vi "combinational-logic-7-segment-origional.vi"(8 "4-bit-reg-input":T1) -> (0 "4-bit-reg-output":T1, 3 "7-segment CTRL out":T2)   [LabVIEW 2021]
uses:
  4-bit-disp.ctl
  7-segment-display.ctl
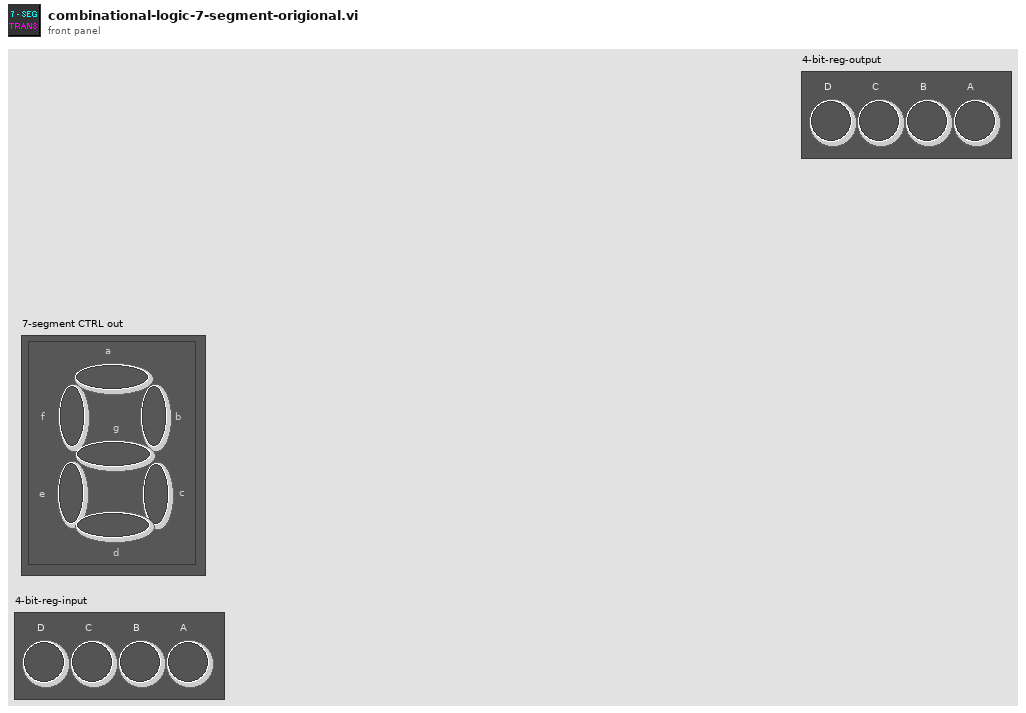
[diagram p1: front panel]
types:
  T1 = typedef "4-bit-disp.ctl" = cluster{"D":bool, "C":bool, "B":bool, "A":bool}
  T2 = typedef "7-segment-display.ctl" = cluster{"a":bool, "b":bool, "c":bool, "d":bool, "e":bool, "f":bool, "g":bool}
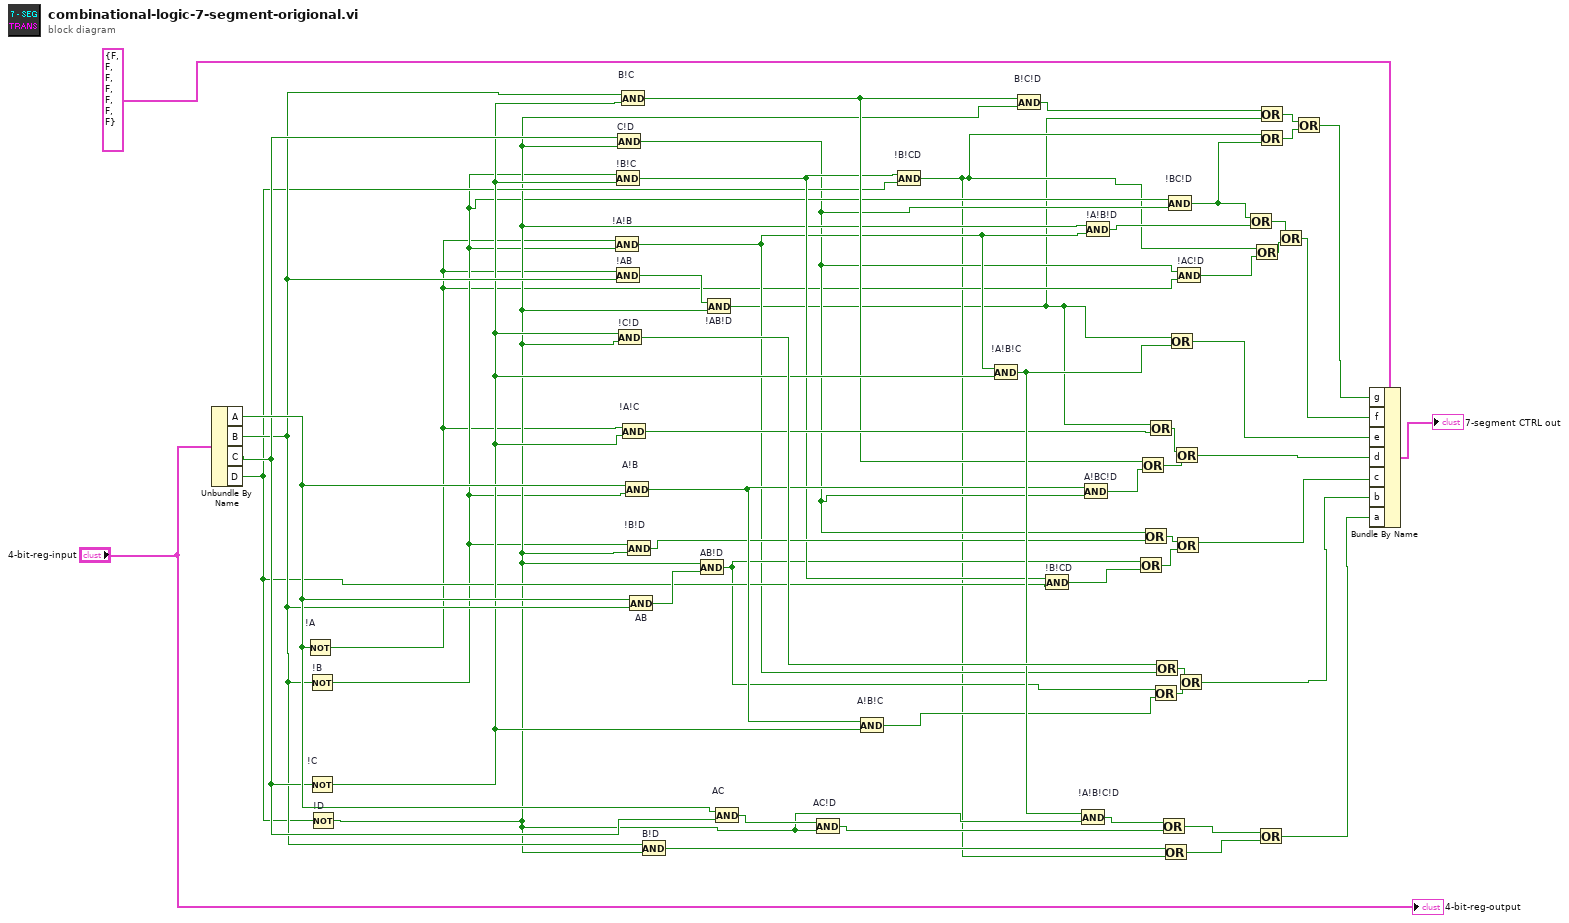
[diagram p0: block diagram]
diagram:
  n1 = Unbundle By Name("4-bit-reg-input") -> ("A"=w36:bool, "B"=w30:bool, "C"=w35:bool, "D"=w19:bool)
  n2 = Not "!A"(x=w36) -> (.not. x?=w7:bool)
  n3 = Not "!B"(x=w30) -> (.not. x?=w10:bool)
  n4 = Not "!C"(x=w35) -> (.not. x?=w28:bool)
  n5 = Not "!D"(x=w19) -> (.not. x?=w12:bool)
  n6 = And "!A!B"(x=w7, y=w10) -> (x .and. y?=w13:bool)
  n7 = And "!B!C"(x=w10, y=w28) -> (x .and. y?=w20:bool)
  n8 = And "!AB"(x=w7, y=w30) -> (x .and. y?=w47:bool)
  n9 = And "C!D"(x=w35, y=w12) -> (x .and. y?=w8:bool)
  n10 = And "!C!D"(x=w28, y=w12) -> (x .and. y?=w38:bool)
  n11 = And "B!C"(x=w30, y=w28) -> (x .and. y?=w26:bool)
  n12 = And "!A!C"(x=w7, y=w28) -> (x .and. y?=w29:bool)
  n13 = And "A!B"(x=w36, y=w10) -> (x .and. y?=w24:bool)
  n14 = And "!B!D"(x=w10, y=w12) -> (x .and. y?=w22:bool)
  n15 = And "AB"(x=w36, y=w30) -> (x .and. y?=w21:bool)
  n16 = And "B!D"(x=w30, y=w12) -> (x .and. y?=w37:bool)
  n17 = And "AB!D"(x=w12, y=w21) -> (x .and. y?=w16:bool)
  n18 = And "!AB!D"(x=w47, y=w12) -> (x .and. y?=w1:bool)
  n19 = And "AC"(x=w36, y=w35) -> (x .and. y?=w33:bool)
  n20 = And "AC!D"(x=w33, y=w12) -> (x .and. y?=w34:bool)
  n21 = And "A!B!C"(x=w24, y=w28) -> (x .and. y?=w15:bool)
  n22 = And "!B!CD"(x=w20, y=w19) -> (x .and. y?=w2:bool)
  n23 = And "!A!B!C"(x=w13, y=w28) -> (x .and. y?=w31:bool)
  n24 = And "B!C!D"(x=w26, y=w12) -> (x .and. y?=w4:bool)
  n25 = And "!B!CD"(x=w20, y=w19) -> (x .and. y?=w17:bool)
  n26 = And "!A!B!C!D"(x=w31, y=w12) -> (x .and. y?=w32:bool)
  n27 = And "A!BC!D"(x=w24, y=w8) -> (x .and. y?=w25:bool)
  n28 = And "!A!B!D"(x=w12, y=w13) -> (x .and. y?=w11:bool)
  n29 = Or(x=w16, y=w17) -> (x .or. y?=w45:bool)
  n30 = Or(x=w26, y=w25) -> (x .or. y?=w27:bool)
  n31 = Or(x=w8, y=w22) -> (x .or. y?=w23:bool)
  n32 = Or(x=w1, y=w29) -> (x .or. y?=w48:bool)
  n33 = Or(x=w16, y=w15) -> (x .or. y?=w43:bool)
  n34 = Or(x=w38, y=w13) -> (x .or. y?=w44:bool)
  n35 = Or(x=w32, y=w34) -> (x .or. y?=w41:bool)
  n36 = Or(x=w37, y=w2) -> (x .or. y?=w40:bool)
  n37 = And "!BC!D"(x=w10, y=w8) -> (x .and. y?=w3:bool)
  n38 = Or(x=w1, y=w31) -> (x .or. y?=w50:bool)
  n39 = Or(x=w48, y=w27) -> (x .or. y?=w49:bool)
  n40 = Or(x=w23, y=w45) -> (x .or. y?=w46:bool)
  n41 = And "!AC!D"(x=w8, y=w7) -> (x .and. y?=w9:bool)
  n42 = Or(x=w44, y=w43) -> (x .or. y?=w18:bool)
  n43 = Or(x=w3, y=w11) -> (x .or. y?=w14:bool)
  n44 = Or(x=w2, y=w9) -> (x .or. y?=w51:bool)
  n45 = Or(x=w41, y=w40) -> (x .or. y?=w42:bool)
  n46 = Or(x=w4, y=w1) -> (x .or. y?=w5:bool)
  n47 = Or(x=w2, y=w3) -> (x .or. y?=w6:bool)
  n48 = Or(x=w14, y=w51) -> (x .or. y?=w52:bool)
  n49 = Or(x=w5, y=w6) -> (x .or. y?=w53:bool)
  n50 = Bundle By Name(cluster=T2 {"a"=FALSE, "b"=FALSE, "c"=FALSE, "d"=FALSE, "e"=FALSE, "f"=FALSE, "g"=FALSE} ("7-seg-typedef"), "g"=w53, "f"=w52, "e"=w50, "d"=w49, "c"=w46, "b"=w18, "a"=w42) -> (→"7-segment CTRL out":T2)
  "4-bit-reg-output" <- "4-bit-reg-input"
